vi "Colors.vi"(2 "Pixels colors (uchar)":u32[](array[numeric]), 3 "stdout":string) -> (13 "Number of Traces":i32, 14 "Corners color (CLUT)":i32, 15 "Corners":u32(colorbox), 16 "Traces":u32[](array[colorbox]), 17 "Traces colors string (RGB)":string[](array[string]), 18 "Traces colors (CLUT)":i32[](array[numeric]), 19 "Traces colors (RGB)":u8[][](array[numeric]))   [LabVIEW 2023]
uses:
  <vilib>/Utility/error.llb/Trim Whitespace One-Sided.vi
panel:
  in  "User interface":T1(tab)
  in  "User entries":enum32{""}(tab)
  in  "Customization":enum32{"Customization"}(tab)
  in  "Colors":enum32{"Colors"}(tab)
  in  "Size":enum32{"Size"}(tab)
  in  "Loop FOR 1":enum32{"Loop FOR 1"}(tab)
  out "appended array":u8[](array[numeric])
  out "Color CLUT at index I":u32
  out "Color Box":u32(colorbox)
  out "B":u8
  out "G":u8
  out "R":u8
  in  "Arrays":enum32{"Arrays"}(tab)
  in  "Script.m":enum32{"Script.m"}(tab)
  in  "Extract.c output string scan":enum32{"Extract.c output string scan"}(tab)
  in  "T: tt1 tt2 tt3 ...":enum32{"T: tt1 tt2 tt3 ..."}(tab)
  out "before substring \"T:\"":string
  out "after substring \"T:\"":string
  in  "C: cc":enum32{"C: cc"}(tab)
  out "string out":string
  in  "Loop FOR 2":enum32{"Loop FOR 2"}(tab)
  out "Array RGB to Array string":string
  in  "LabVIEW":enum32{"LabVIEW"}(tab)
  in  "MATLAB":enum32{"MATLAB"}(tab)
  in  "C":enum32{"C"}(tab)
  in  "MATLAB":enum32{"MATLAB"}(tab)
  in  "C":enum32{"C"}(tab)
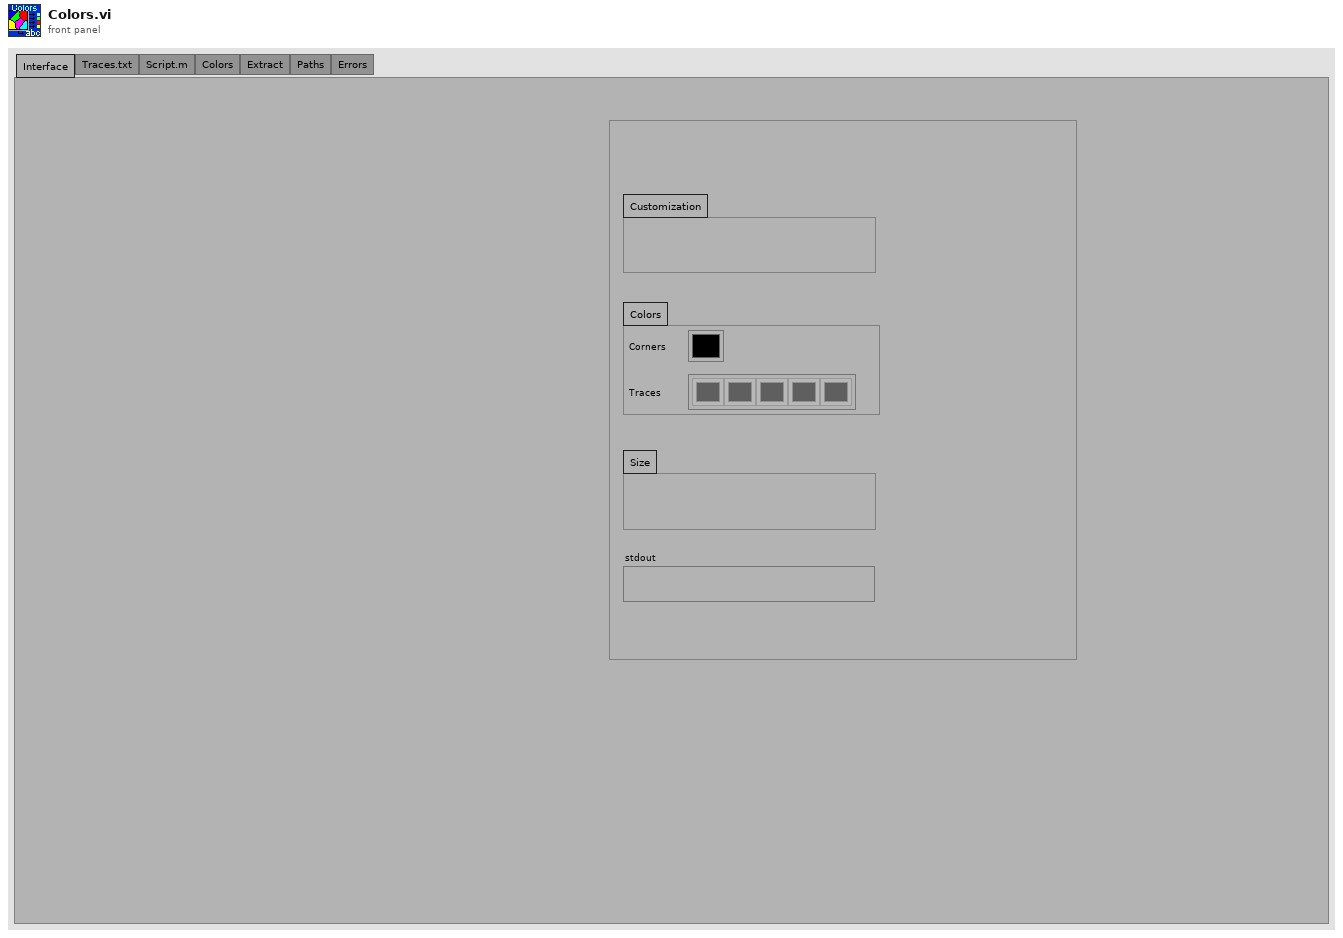
[diagram p1: front panel]
types:
  T1 = enum32{"Interface", "Traces.txt", "Script.m", "Colors", "Extract", "Paths", "Errors"}
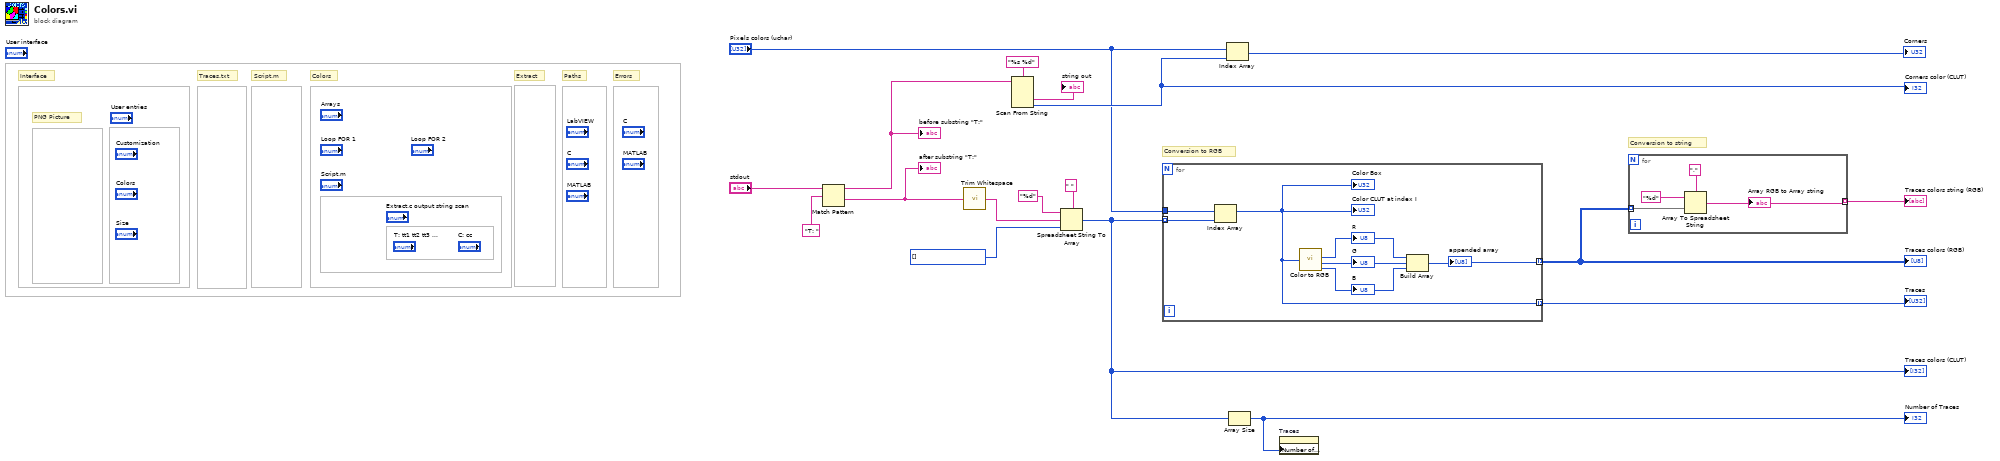
[diagram p0: block diagram]
diagram:
  # "Conversion to RGB"
  # "Conversion to string"
  # "PNG Picture"
  # "Errors"
  # "Paths"
  # "Extract"
  # "Colors"
  # "Script.m"
  # "Traces.txt"
  # "Interface"
  n1 = Match Pattern(string="stdout", regular expression="T: ") -> (before substring=w13:string, after substring=w10:string)  [unwired: 1 in, 2 out]
  "after substring \"T:\"" <- w10
  "before substring \"T:\"" <- w13
  n2 = call <vilib>:"Trim Whitespace.vi"("string"=w10) -> ("trimmed string"=w9:string)  [unwired: 1 in]
  n3 = Scan From String(format string="%s %d", input string=w13) -> (output 1=→"string out":string, output 2=w17:i32)  [unwired: 4 in, 3 out]
  "Corners color (CLUT)" <- w17
  n4 = Spreadsheet String To Array(delimiter (Tab)=" ", format string="%d", spreadsheet string=w9, array type (2D Dbl)=i32[] []) -> (array=w7:i32[])
  "Traces colors (CLUT)" <- w7
  n5 = for {
    tunnel: w7 -> [w25] mode=indexing
    tunnel: "Pixels colors (uchar)" -> [w24]
    tunnel: [w23] -> w8 mode=indexing
    tunnel: [w19] -> w5 mode=indexing
    n6 = Index Array(array=w24, index=w25) -> (element=w23:u32)
    "Color CLUT at index I" <- w23
    "Color Box" <- w23
    n7 = call <vilib>:"Color to RGB.vi"("Color"=w23) -> ("R"=w22:u8, "G"=w21:u8, "B"=w20:u8)  [unwired: 1 out]
    "R" <- w22
    "G" <- w21
    "B" <- w20
    n8 = Build Array(w22, w21, w20) -> (w19:u8[])
    "appended array" <- w19
  }
  "Traces" <- w8
  "Traces colors (RGB)" <- w5
  n9 = Index Array(array="Pixels colors (uchar)", index=w17) -> (element=→"Corners":u32)
  n10 = Array Size(array=w7) -> (size(s)=w6:i32)
  "Number of Traces" <- w6
  n11 = property on="Traces" class="Arr (strict)"("Number of Columns"=w6) -> ()  [unwired: 2 in, 2 out]
  n12 = for {
    tunnel: w5 -> [w29] mode=indexing
    tunnel: [w26] -> w4 mode=indexing
    n13 = Array To Spreadsheet String(delimiter (Tab)=",", array=w29, 3:"%d" ("format string")) -> (spreadsheet string=w26:string)
    "Array RGB to Array string" <- w26
  }
  "Traces colors string (RGB)" <- w4
